vi "Test_ServiceDoesnot_Exist.vi"() -> (0 "Array of Error Description":T1)   [LabVIEW 2022 SP3]
uses:
  gRPC_ATS/TestUtility/utility.llb/array of error description.ctl
  gRPC_ATS/TestUtility/utility.llb/error description.ctl
  gRPC_ATS/TestUtility/utility.llb/error type.ctl
panel:
  out "Pass":bool
  in  "Server VI path":path
  in  "error in":errorcluster
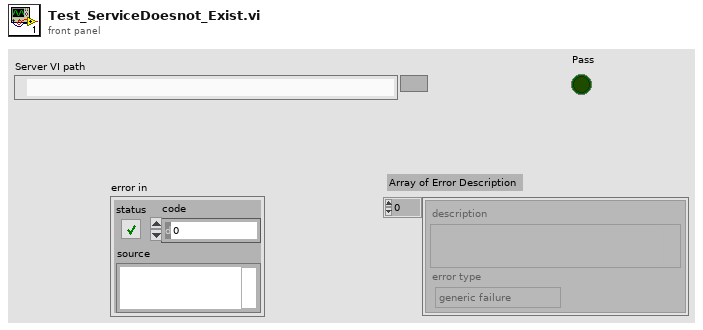
[diagram p1: front panel]
types:
  T1 = typedef "array of error description.ctl" = T2[]
  T2 = typedef "error description.ctl" = cluster{"description":string, "error type":T3}
  T3 = typedef "error type.ctl" = enum32{"generic failure", "boundary case", "precision", "expected error"}
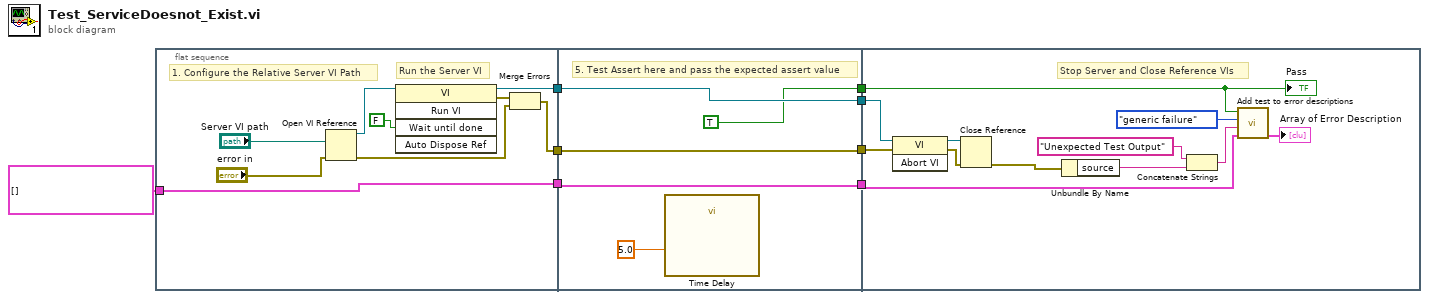
[diagram p0: block diagram]
diagram:
  n1 = flat-sequence {
    tunnel: T1 [] ("error descriptions in") -> [w13]
    tunnel: [w13] -> w3
    tunnel: [w12] -> w2
    tunnel: [w9] -> w1
    tunnel: w3 -> [w22]
    tunnel: [w22] -> w8
    tunnel: [w19] -> w7
    tunnel: [w21] -> w6
    tunnel: w2 -> [w21]
    tunnel: [TRUE] -> w4
    tunnel: w1 -> [w19]
    tunnel: w8 -> [w29]
    tunnel: w7 -> [w25]
    tunnel: w6 -> [w26]
    tunnel: w4 -> [w24]
    frame #0 {
      # "1. Configure the Relative Server VI Path"
      # "Run the Server VI"
      n2 = Open VI Reference(vi path="Server VI path", error in (no error)="error in") -> (vi reference=w15:refnum<vi>, error out=w11:errorcluster)  [unwired: 4 in]
      n3 = invoke class="VI" method="Run VI"(reference=w15, "Wait until done"=FALSE ("Wait Until Done")) -> (reference out=w12:refnum<vi>, error out=w10:errorcluster)  [unwired: 3 in, 3 out]
      n4 = Merge Errors(w10, w11) -> (w9:errorcluster)
    }
    frame #1 {
      # "5. Test Assert here and pass the expected assert value"
      n5 = call "Time Delay"("Delay Time (s)"=5.0) -> ()  [unwired: 10 in, 1 out]
    }
    frame #2 {
      # "Stop Server and Close Reference VIs"
      n6 = invoke class="VI" method="Abort VI"(reference=w26, error in=w25) -> (reference out=w27:refnum<vi>, error out=w28:errorcluster)  [unwired: 1 in, 1 out]
      n7 = Close Reference(reference=w27, error in (no error)=w28) -> (error out=w23:errorcluster)
      n8 = Unbundle By Name(w23) -> ("source"=w31:string)
      n9 = Concatenate Strings("Unexpected Test Output" ("string"), w31) -> (w32:string)
      n10 = call "Add test to error descriptions.vi"("error descriptions in"=w29, "error string"=w32, "error type"=error_type."generic failure", "pass"=w24) -> ("error description out"=→"Array of Error Description":T1)  [unwired: 3 in]
      "Pass" <- w24
    }
  }
